vi "Handle Command.vi"(8 "error in":errorcluster, 10 "Change Laser Vrange in":refnum<class "Change Laser Modulation.lvclass">, 11 "Object In":refnum<class>) -> (0 "error out":errorcluster, 1 "Command Successful?":bool, 2 "Change Laser Vrange out":refnum<class "Change Laser Modulation.lvclass">, 3 "Object Out":refnum<class>)   [LabVIEW 2014, in "ePAS Library.lvlib" / "Change Laser Modulation.lvclass"]
doc: "Abstract method for accomplishing the execution of a command directed to an instrument object on the wire."
uses:
  Change Laser Modulation.lvclass
  Instrument/ePAS.lvclass
  Instrument/ePAS.lvclass/ePAS.ctl
  Change Laser Modulation.lvclass/Change Laser Modulation.ctl
  reusable/Instrument/Instrument.lvclass/Instrument.ctl
  reusable/Instrument/Read ExtCom.vi
  reusable/Instrument/Read Log Session.vi
  <vilib>/Utility/error.llb/Error Cluster From Error Code.vi
  <vilib>/rvi/errors/niLvFpgaAdjustHostInterfaceError.vi
  <userlib>/_Session Fwk/Session - Root.lvclass
  <vilib>/rvi/interface/nirviReadWriteControl/nirviReadWriteControl.xnode
  FPGA/R FPGA Ref.ctl
  FPGA Bitfiles/FPGAServerV2.lvbitx
  FPGA/Session/Exscalabar FPGA.lvclass
  ePAS Library.lvlib
  reusable/Session APIs/Session Log/System Log.lvclass
  NiFpgaLv.dll
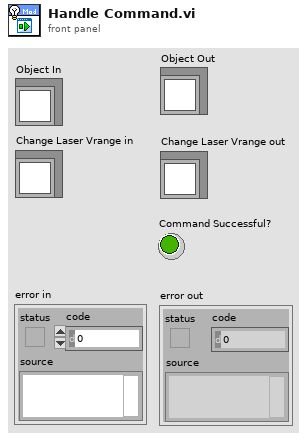
[diagram p1: front panel]
types:
  T1 = typedef "Session - Root.lvclass/Session Handle.ctl" = refnum<data-value>
  T2 = typedef "ePAS Library.lvlib/R FPGA Ref.ctl" = refnum<k20>
  T3 = cluster{"f0":fxp<+,32,0>, "Scale":fxp<+,32,0>, "Offset":i16, "Mod":enum8{"Sine", "Square"}}
  T4 = cluster{"f0":fxp<+,32,0>, "Scale":fxp<+,32,0>, "Offset":i16, "Mod":enum8{"Sine", "Square"}}[]
  T5 = cluster{"tag":string, "section":string, "data":variant}
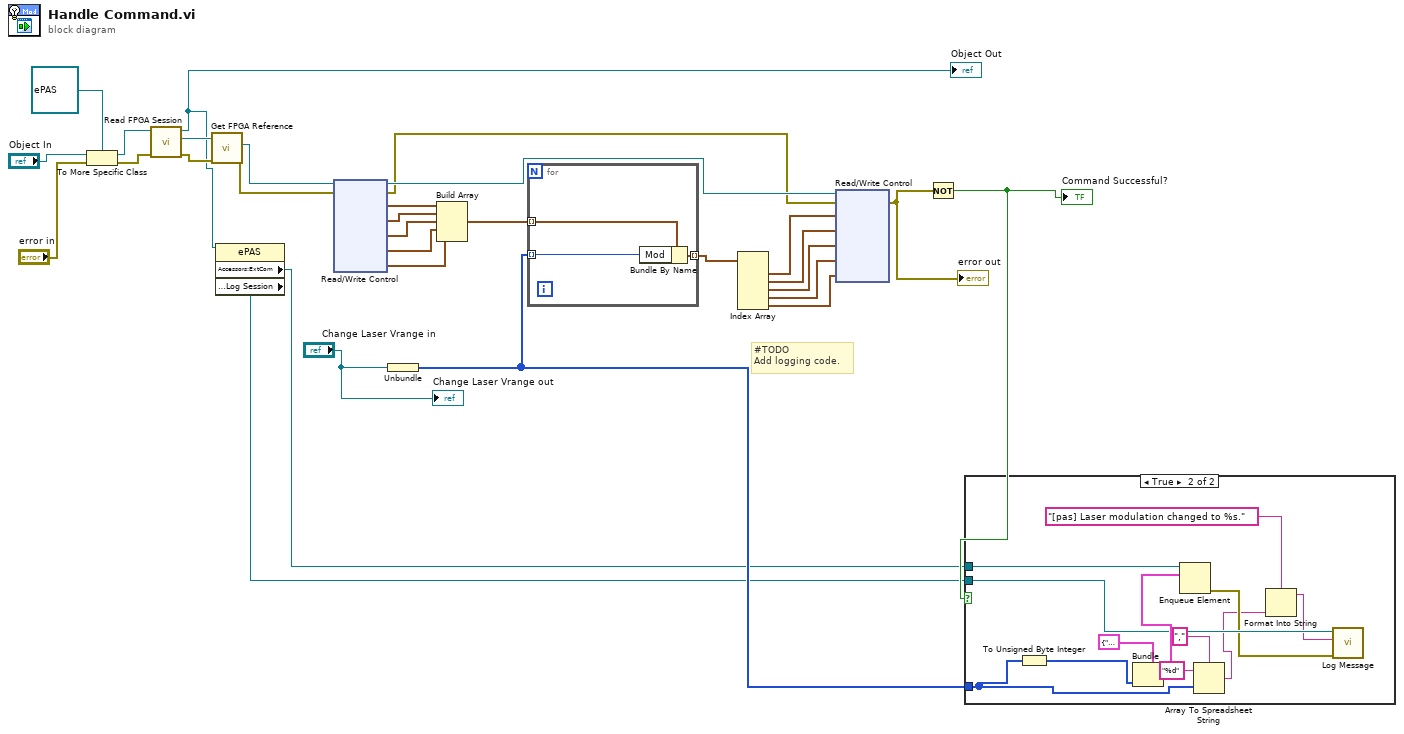
[diagram p0: block diagram]
diagram:
  # "#TODO\nAdd logging code."
  n1 = To More Specific Class(target class=refnum<class "ePAS.lvclass"> refnum ("ePAS"), reference="Object In", error in="error in") -> (specific class reference=w28:refnum<class "ePAS.lvclass">, error out=w27:errorcluster)
  n2 = call "Read FPGA Session.vi"("error in (no error)"=w27, "ePAS in"=w28) -> ("error out"=w10:errorcluster, "Session Handle"=w26:T1, "ePAS out"=w3:refnum<class "ePAS.lvclass">)  [unwired: 7 in]
  "Object Out" <- w3
  n3 = call "Get FPGA Reference.vi"("error in"=w10, "Session In"=w26) -> ("error out"=w8:errorcluster, "Ex FPGA Ref"=w25:T2)  [unwired: 7 in, 1 out]
  n4 = property class="ePAS"(reference=w3) -> ("Accessors:ExtCom"=w2:refnum<queue>, "Accessors:Log Session"=w1:T1)  [unwired: 1 in, 2 out]
  n5 = xnode "Read/Write Control"("FPGA VI Reference In"=w25, "error in"=w8) -> ("FPGA VI Reference Out"=w18:T2, "error out"=w17:errorcluster, "Cell 1"=w24:T3, "Cell 2"=w23:T3, "Cell 3"=w22:T3, "Cell 4"=w21:T3, "Cell 5"=w20:T3)
  n6 = Unbundle("Change Laser Vrange in") -> (w4:enum8{"Sine", "Square"}[])
  n7 = Build Array(w24, w23, w22, w21, w20) -> (w19:T4)
  n8 = for {
    tunnel: w19 -> [w33] mode=indexing
    tunnel: w4 -> [w31] mode=indexing
    tunnel: [w32] -> w16 mode=indexing
    n9 = Bundle By Name(cluster=w33, "Mod"=w31) -> (w32:T3)
  }
  n10 = Index Array(array=w16) -> (element #1=w15:T3, element #2=w14:T3, element #3=w13:T3, element #4=w12:T3, element #5=w11:T3)  [unwired: 5 in]
  n11 = xnode "Read/Write Control"("FPGA VI Reference In"=w18, "error in"=w17, "Cell 1"=w15, "Cell 2"=w14, "Cell 3"=w13, "Cell 4"=w12, "Cell 5"=w11) -> ("error out"=w7:errorcluster)  [unwired: 1 out]
  "error out" <- w7
  n12 = Not(x=w7) -> (.not. x?=w5:bool)
  "Command Successful?" <- w5
  n13 = case shown="True" w5 {
    tunnel: w2 -> [_ w45]
    tunnel: w4 -> [_ w35]
    tunnel: w1 -> [_ w42]
    frame False {
    }
    frame True {
      n14 = To Unsigned Byte Integer(number=w35) -> (unsigned 8bit integer=w34:u8[])
      n15 = Bundle(cluster=T5 {"tag"="modulation", "section"="pas.las", "data"=variant} ("element"), "data"=w34) -> (w43:T5)  [unwired: 2 in]
      n16 = Enqueue Element(queue=w45, element=w43) -> (error out=w39:errorcluster)  [unwired: 2 in, 2 out]
      n17 = Array To Spreadsheet String(delimiter (Tab)=",", array=w35, 3:"%d" ("format string")) -> (spreadsheet string=w37:string)
      n18 = Format Into String(format string="[pas] Laser modulation changed to %s.", w37) -> (resulting string=w40:string)  [unwired: 2 in, 1 out]
      n19 = call "Log Message.vi"("error in"=w39, "MSG In"=w40, "session in"=w42) -> ()  [unwired: 7 in, 2 out]
    }
  }
  "Change Laser Vrange out" <- "Change Laser Vrange in"
